vi "SizeUp.vi"() -> ()   [LabVIEW 2024, in "RefTypedCircularBuffer.Tests.Units.lvlib"]
uses:
  RefTypedCircularBuffer.Tests.Units.lvlib
  <vilib>/addons/_JKI Toolkits/Caraya/classes/Assert/Assert.lvclass
  <vilib>/addons/_JKI Toolkits/Caraya/classes/Assert/Assert True.vi
  <vilib>/addons/_JKI Toolkits/Caraya/classes/Assert/Assert Equal Value and Type_Variant.vi
  <vilib>/addons/_JKI Toolkits/Caraya/classes/Assert/Assert False.vi
  <vilib>/addons/_JKI Toolkits/Caraya/classes/Test/Test.lvclass
  RefTypedCircularBuffer.lvclass
  <vilib>/addons/_JKI Toolkits/Caraya/classes/Assert/Assert Equal Value_Variant.vi
  TypedCircularBuffer/Type.ctl
  TypedCircularBuffer/TypedCircularBuffer.lvclass
  Type.ctl
panel:
  out "Copied Buffer 3":T1[](array[typedef])
  out "Copied Buffer 2":T1[](array[typedef])
  out "Full?":bool
  out "Copied Buffer":T1[](array[typedef])
  in  "Size up Add Expected":T2[](array[typedef])=[0, 1, 2, 3, 4, 5, 6, 7, 8, 9, 255]
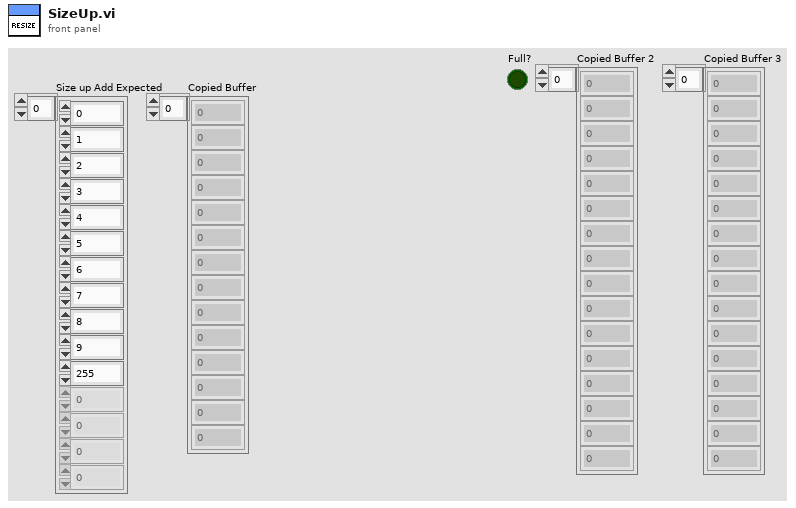
[diagram p1: front panel]
types:
  T1 = typedef "RefTypedCircularBuffer.lvclass/Type.ctl" = u8
  T2 = typedef "TypedCircularBuffer.lvclass/Type.ctl" = i32
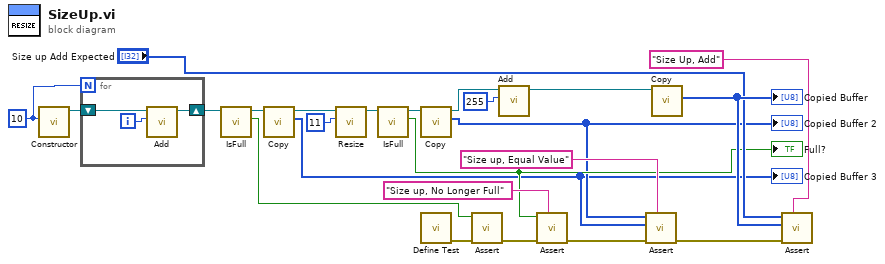
[diagram p0: block diagram]
diagram:
  w16 = u32 10 ("Capacity")
  n1 = call "Constructor.vi"("Capacity"=w16) -> ("TypedCircularBuffer out"=w17:refnum<class "RefTypedCircularBuffer.lvclass">)  [unwired: 10 in]
  n2 = for {
    N: w16 -> [_]
    shift-right: [w26] -> w10
    shift-left: w17 -> [w27]
    i -> [w25]
    n3 = call "Add.vi"("Element"=w25, "TypedCircularBuffer in"=w27) -> ("TypedCircularBuffer out"=w26:refnum<class "RefTypedCircularBuffer.lvclass">)  [unwired: 7 in, 2 out]
  }
  n4 = call "IsFull.vi"("TypedCircularBuffer in"=w10) -> ("Full?"=w9:bool, "TypedCircularBuffer out"=w1:refnum<class "RefTypedCircularBuffer.lvclass">)  [unwired: 9 in]
  n5 = call "Copy.vi"("TypedCircularBuffer in"=w1) -> ("Copied Buffer"=w2:T1[], "TypedCircularBuffer out"=w15:refnum<class "RefTypedCircularBuffer.lvclass">)  [unwired: 9 in]
  "Copied Buffer 3" <- w2
  n6 = call "Resize.vi"("Capacity"=u32 11, "TypedCircularBuffer in"=w15) -> ("TypedCircularBuffer out"=w4:refnum<class "RefTypedCircularBuffer.lvclass">)  [unwired: 9 in]
  n7 = call "IsFull.vi"("TypedCircularBuffer in"=w4) -> ("Full?"=w6:bool, "TypedCircularBuffer out"=w5:refnum<class "RefTypedCircularBuffer.lvclass">)  [unwired: 9 in]
  "Full?" <- w6
  n8 = call "Copy.vi"("TypedCircularBuffer in"=w5) -> ("Copied Buffer"=w3:T1[], "TypedCircularBuffer out"=w13:refnum<class "RefTypedCircularBuffer.lvclass">)  [unwired: 9 in]
  "Copied Buffer 2" <- w3
  n9 = call <vilib>:"Define Test.vi"() -> ("error out"=w19:errorcluster)  [unwired: 10 in, 1 out]
  n10 = call-poly <vilib>:"Assert.vi"("error in (no error)"=w19, "True?"=w9) -> ("error out"=w24:errorcluster)  [unwired: 8 in, 1 out]
  n11 = call "Add.vi"("Element"=u8 255, "TypedCircularBuffer in"=w13) -> ("TypedCircularBuffer out"=w11:refnum<class "RefTypedCircularBuffer.lvclass">)  [unwired: 7 in, 2 out]
  n12 = call-poly <vilib>:"Assert.vi"("Label"="Size up, No Longer Full", "error in (no error)"=w24, "False?"=w6) -> ("error out"=w23:errorcluster)  [unwired: 7 in, 1 out]
  n13 = call-poly <vilib>:"Assert.vi"("Label"="Size up, Equal Value", "error in (no error)"=w23, "Y"=w2, "X"=w3) -> ("error out"=w18:errorcluster)  [unwired: 6 in, 1 out]
  n14 = call "Copy.vi"("TypedCircularBuffer in"=w11) -> ("Copied Buffer"=w8:T1[])  [unwired: 9 in, 1 out]
  "Copied Buffer" <- w8
  n15 = call-poly <vilib>:"Assert.vi"("Label"="Size Up, Add", "error in (no error)"=w18, "Y"=w8, "X"="Size up Add Expected") -> ()  [unwired: 6 in, 2 out]
